vi "Script_Create Steering Frame.vi"(6 "error source terminal refnum":refnum<vi>, 8 "error in (no error)":errorcluster, 10 "owner diagram refnum":refnum<vi>, 11 "steering frame in":refnum<class "NI_Robotics_Steering Frame.lvclass">) -> (0 "error out":errorcluster, 1 "created?":bool, 2 "steering frame out terminal refnum":refnum<vi>, 3 "steering frame out":refnum<class "NI_Robotics_Steering Frame.lvclass">, 4 "error out terminal refnum":refnum<vi>)   [LabVIEW 2017, in "NI_Robotics_Scripting Utilities.lvlib"]
uses:
  <vilib>/robotics/Utilities/Scripting/NI_Robotics_Scripting Utilities.lvlib
  <vilib>/robotics/Steering/Steering Frame/NI_Robotics_Steering Frame.lvclass
  <vilib>/robotics/Steering/Steering Frame/NI_Robotics_Steering Frame.lvclass/NI_Robotics_Steering Frame.ctl
  <vilib>/robotics/Steering/Steering Frame/Get Multiple Wheels in Steering Frame.vi
  <vilib>/robotics/Utilities/Scripting/Script_Create Omnidirectional Wheel.vi
  <vilib>/robotics/Utilities/Scripting/Script_Create Mecanum Wheel.vi
  <vilib>/robotics/Utilities/Scripting/Script_Create Caster Wheel.vi
  <vilib>/robotics/Utilities/Scripting/Script_Create Steering Wheel.vi
  <vilib>/robotics/Utilities/Scripting/Script_Create Fixed Wheel.vi
  <vilib>/robotics/Utilities/Scripting/Script_Create Steering Frame_Mecanum.vi
  <vilib>/robotics/Utilities/Scripting/Script_Create Steering Frame_Ackermann.vi
  <vilib>/robotics/Utilities/Scripting/Script_Create Steering Frame_Differential.vi
  <vilib>/robotics/Utilities/Scripting/Script_Create Steering Frame_User Defined.vi
  <vilib>/robotics/Steering/Wheel/NI_Robotics_Wheel.lvclass
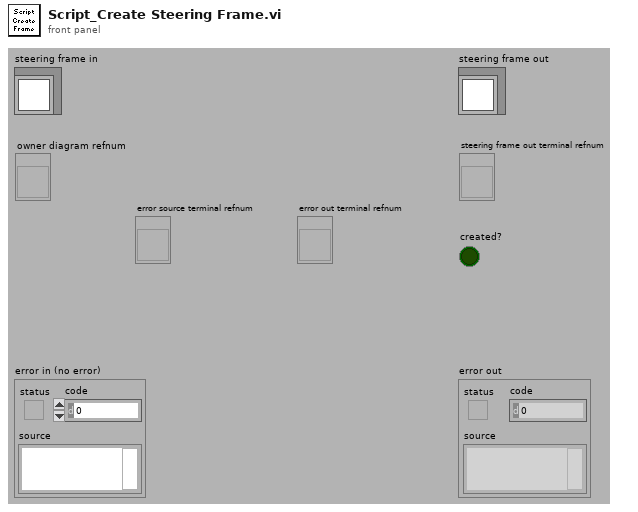
[diagram p1: front panel]
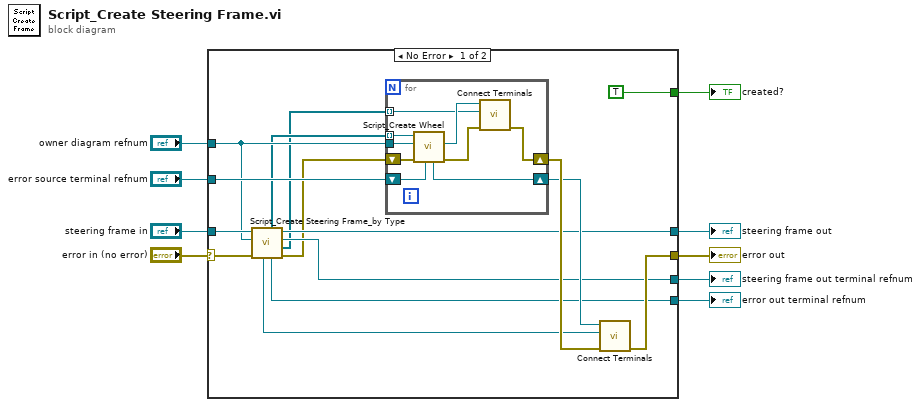
[diagram p0: block diagram]
diagram:
  n1 = case shown="No Error" "error in (no error)" {
    selector: "error in (no error)" -> [w11 w35]
    tunnel: [w21 w35] -> w8
    tunnel: [w17 w34] -> w6
    tunnel: "steering frame in" -> [w19 w34]
    tunnel: "owner diagram refnum" -> [w18 _]
    tunnel: "error source terminal refnum" -> [w23 _]
    tunnel: [w13 _] -> w3
    tunnel: [TRUE _] -> w2
    tunnel: [w15 _] -> w1
    frame No Error {
      n2 = call <vilib>:"Script_Create Steering Frame_by Type.vi"("error in (no error)"=w11, "owner diagram refnum"=w18, "steering frame in"=w19) -> ("error out"=w10:errorcluster, "bundler input terminal refnums"=w14:refnum<vi>[], "steering frame out terminal refnum"=w15:refnum<vi>, "steering frame out"=w17:refnum<class "NI_Robotics_Steering Frame.lvclass">, "error out terminal refnum"=w13:refnum<vi>, "wheels"=w16:refnum<class "NI_Robotics_Wheel.lvclass">[], "error in terminal refnum"=w12:refnum<vi>)  [unwired: 2 in]
      n3 = for {
        tunnel: w16 -> [w33] mode=indexing
        shift-right: [w27] -> w24
        shift-left: w10 -> [w32]
        tunnel: w18 -> [w31]
        shift-right: [w28] -> w22
        shift-left: w23 -> [w29]
        tunnel: w14 -> [w26] mode=indexing
        n4 = call <vilib>:"Script_Create Wheel.vi"("error source terminal refnum"=w29, "error in (no error)"=w32, "owner diagram refnum"=w31, "wheel in"=w33) -> ("error out"=w25:errorcluster, "wheel out terminal refnum"=w30:refnum<vi>, "error out terminal refnum"=w28:refnum<vi>)  [unwired: 4 in, 1 out]
        n5 = call <vilib>:"Connect Terminals.vi"("error in (no error)"=w25, "sink terminal"=w26, "source terminal"=w30) -> ("error out"=w27:errorcluster)  [unwired: 7 in, 1 out]
      }
      n6 = call <vilib>:"Connect Terminals.vi"("error in (no error)"=w24, "sink terminal"=w12, "source terminal"=w22) -> ("error out"=w21:errorcluster)  [unwired: 7 in, 1 out]
    }
    frame Error {
    }
  }
  "error out" <- w8
  "steering frame out" <- w6
  "steering frame out terminal refnum" <- w1
  "error out terminal refnum" <- w3
  "created?" <- w2
